vi "Polygraph.vi"() -> ()   [LabVIEW 2018]
uses:
  <vilib>/Instr/_visa.llb/VISA Configure Serial Port (Instr).vi
panel:
  in  "Baseline pulse":dbl
  in  "Baseline Humid.":dbl
  in  "Baseline Temp.":dbl
  in  "Ask question":bool
  out "LIE":bool
  out "INCONCLUSIVE":bool
  out "TRUTH":bool
  out "Humidity":dbl(knob) scale=0.0..100.0
  out "Body Temperature":dbl(slide) scale=0.0..100.0
  out "Body Temperature (C)":dbl
  out "Humidity (%)":dbl
  in  "Arduino port":refnum<visa-resource-name>
  in  "Stop":bool
  out "Heartbeat Sensor Data":dbl
  in  "Heartbeat sound path":path
  out "Heartbeat Chart":dbl[](graph)
  # "Pulse"
  # "Skin humidity"
  # "Body Temperature"
  # "Controls"
  # "Polygraph"
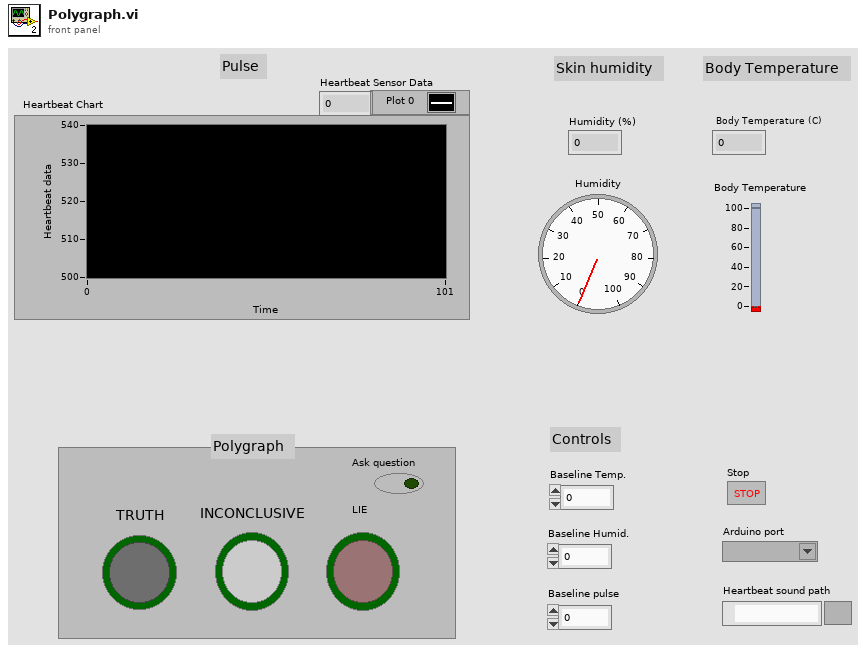
[diagram p1: front panel]
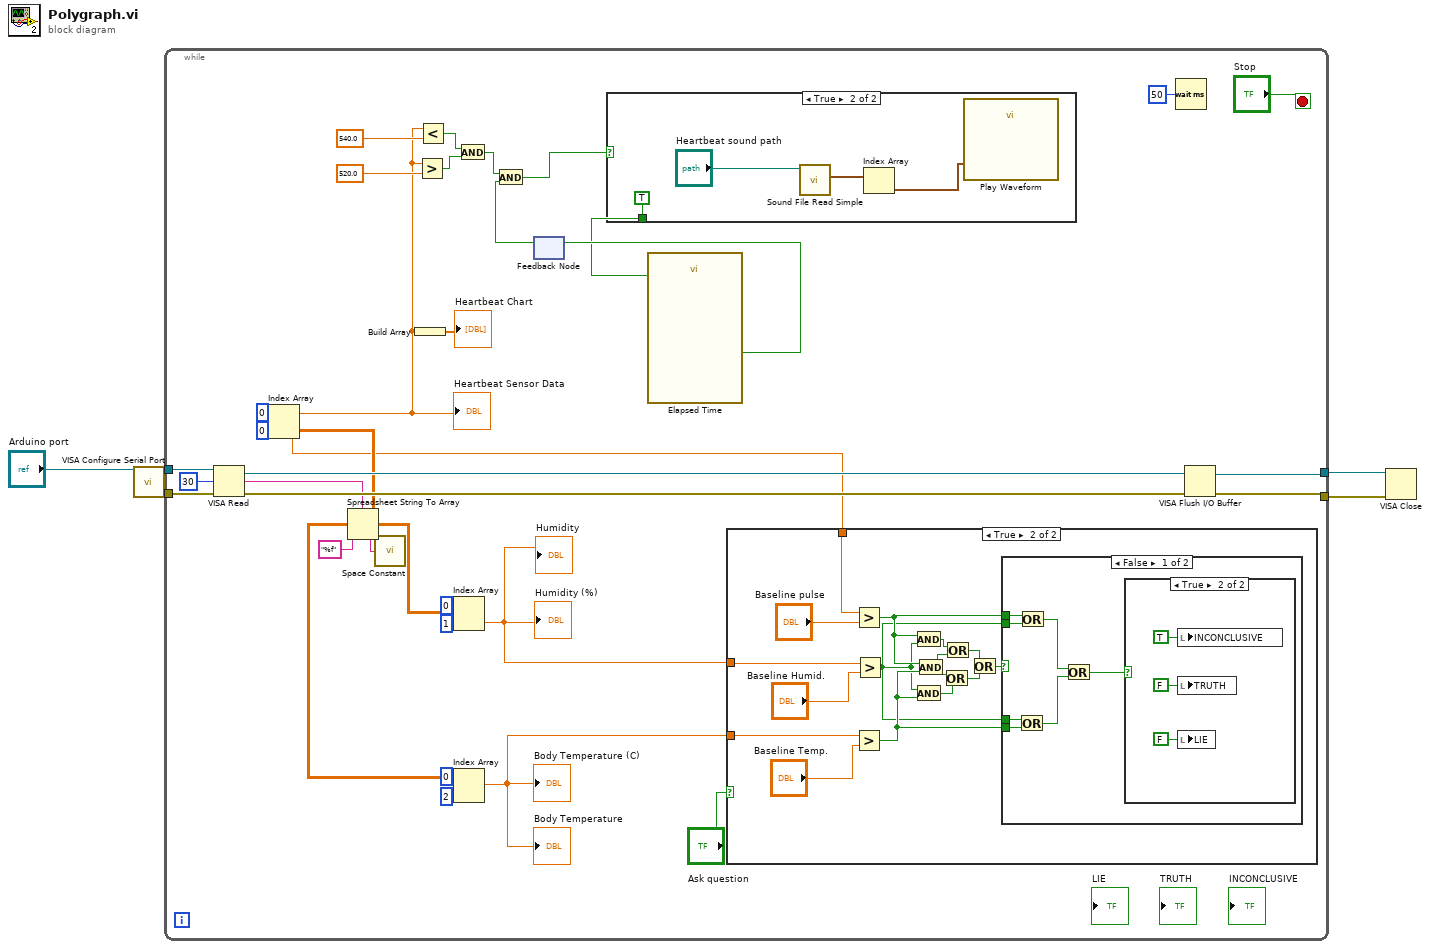
[diagram p0: block diagram]
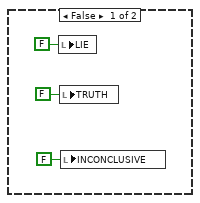
[diagram p2: hidden frame]
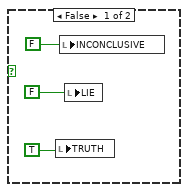
[diagram p3: hidden frame]
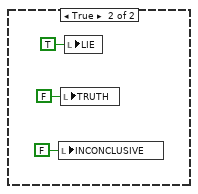
[diagram p4: hidden frame]
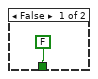
[diagram p5: hidden frame]
diagram:
  n1 = call-poly "VISA Configure Serial Port"("VISA resource name"="Arduino port") -> ("VISA resource name out"=w4:refnum<visa-resource-name>, "error out"=w3:errorcluster)  [unwired: 13 in]
  n2 = while {
    tunnel: w4 -> [w15]
    tunnel: w3 -> [w14]
    tunnel: [w13] -> w2
    tunnel: [w12] -> w1
    stop <- "Stop" stop-if-true
    n3 = VISA Read(VISA resource name=w15, byte count=u32 30, error in (no error)=w14) -> (VISA resource name out=w26:refnum<visa-resource-name>, read buffer=w16:string, error out=w25:errorcluster)  [unwired: 1 out]
    n4 = call <vilib>:"Space Constant.vi"() -> ("String"=w11:string)
    n5 = Spreadsheet String To Array(delimiter (Tab)=w11, format string="%f", spreadsheet string=w16) -> (array=w10:dbl[][])  [unwired: 1 in]
    n6 = Index Array(array=w10, index (row)=0, index (col)=0 ("disabled index (col)")) -> (element=w8:dbl)
    "Heartbeat Sensor Data" <- w8
    n7 = Build Array(w8) -> (→"Heartbeat Chart":dbl[])
    n8 = Greater?(x=w8, y=520.0) -> (0:w34:bool)
    n9 = Less?(x=w8, y=540.0) -> (x < y?=w33:bool)
    n10 = Index Array(array=w10, index (row)=0, index (col)=1 ("disabled index (col)")) -> (element=w6:dbl)
    "Humidity (%)" <- w6
    "Humidity" <- w6
    n11 = Index Array(array=w10, index (row)=0, index (col)=2 ("disabled index (col)")) -> (element=w7:dbl)
    "Body Temperature (C)" <- w7
    "Body Temperature" <- w7
    n12 = And(x=w33, y=w34) -> (x .and. y?=w31:bool)
    n13 = feedback #1() -> (w28:bool)  [unwired: 1 in]
    n14 = And(x=w31, y=w28) -> (x .and. y?=w30:bool)
    n15 = case shown="True" w30 {
      tunnel: [FALSE TRUE] -> w27
      frame False {
      }
      frame True {
        n16 = call <vilib>:"Sound File Read Simple.vi"("path"="Heartbeat sound path") -> ("data"=w76:waveform(dbl)[])  [unwired: 7 in, 3 out]
        n17 = Index Array(array=w76) -> (element=w75:waveform(dbl))  [unwired: 1 in]
        n18 = call "Play Waveform"("Data"=w75) -> ()  [unwired: 18 in, 1 out]
      }
    }
    n19 = call "Elapsed Time"("Reset"=w27) -> ("Time has Elapsed"=w29:bool)  [unwired: 11 in, 7 out]
    n20 = feedback-in #1(w29) -> ()
    n21 = case shown="True" "Ask question" {
      tunnel: w8 -> [_ w56]
      tunnel: w7 -> [_ w55]
      tunnel: w6 -> [_ w54]
      frame False {
        n22 = local write "LIE"(FALSE ("LIE")) -> ()
        n23 = local write "TRUTH"(FALSE ("TRUTH")) -> ()
        n24 = local write "INCONCLUSIVE"(FALSE ("INCONCLUSIVE")) -> ()
      }
      frame True {
        n25 = Greater?(x=w56, y="Baseline pulse") -> (0:w46:bool)
        n26 = Greater?(x=w55, y="Baseline Temp.") -> (0:w47:bool)
        n27 = Greater?(x=w54, y="Baseline Humid.") -> (0:w45:bool)
        n28 = And(x=w46, y=w45) -> (x .and. y?=w52:bool)
        n29 = And(x=w45, y=w47) -> (x .and. y?=w50:bool)
        n30 = And(x=w46, y=w47) -> (x .and. y?=w51:bool)
        n31 = Or(x=w51, y=w50) -> (x .or. y?=w49:bool)
        n32 = Or(x=w52, y=w51) -> (x .or. y?=w48:bool)
        n33 = Or(x=w48, y=w49) -> (x .or. y?=w53:bool)
        n34 = case shown="False" w53 {
          tunnel: w46 -> [w63 _]
          tunnel: w45 -> [w62 _]
          tunnel: w45 -> [w61 _]
          tunnel: w47 -> [w60 _]
          frame False {
            n35 = Or(x=w61, y=w60) -> (x .or. y?=w58:bool)
            n36 = Or(x=w63, y=w62) -> (x .or. y?=w59:bool)
            n37 = Or(x=w59, y=w58) -> (x .or. y?=w57:bool)
            n38 = case shown="True" w57 {
              frame False {
                n39 = local write "TRUTH"(TRUE) -> ()
                n40 = local write "INCONCLUSIVE"(FALSE ("INCONCLUSIVE")) -> ()
                n41 = local write "LIE"(FALSE ("LIE")) -> ()
              }
              frame True {
                n42 = local write "INCONCLUSIVE"(TRUE ("INCONCLUSIVE")) -> ()
                n43 = local write "TRUTH"(FALSE ("TRUTH")) -> ()
                n44 = local write "LIE"(FALSE ("LIE")) -> ()
              }
            }
          }
          frame True {
            n45 = local write "INCONCLUSIVE"(FALSE ("INCONCLUSIVE")) -> ()
            n46 = local write "TRUTH"(FALSE ("TRUTH")) -> ()
            n47 = local write "LIE"(TRUE ("LIE")) -> ()
          }
        }
      }
    }
    n48 = Wait (ms)(milliseconds to wait=u32 50) -> ()  [unwired: 1 out]
    n49 = VISA Flush I/O Buffer(VISA resource name=w26, error in (no error)=w25) -> (VISA resource name out=w12:refnum<visa-resource-name>, error out=w13:errorcluster)  [unwired: 1 in]
  }
  n50 = VISA Close(VISA resource name=w1, error in (no error)=w2) -> ()  [unwired: 1 out]
